vi "WS1021 MEMS Only 24DUT CV Sweep Header BCBE.vi"(8 "Error In":errorcluster) -> (0 "Error Out":errorcluster, 3 "Name Calculated Header":string[](array[string]))   [LabVIEW 2017]
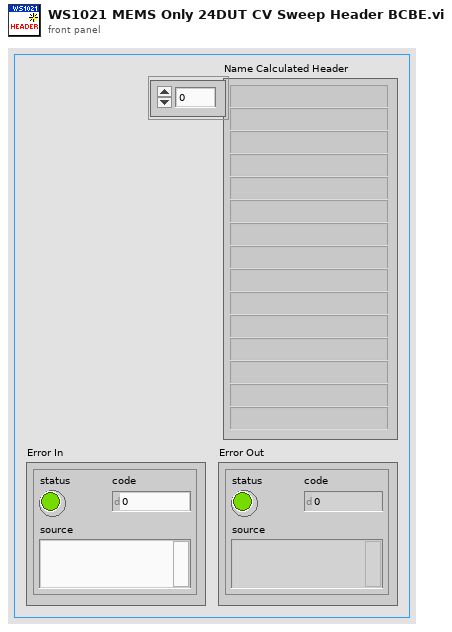
[diagram p1: front panel]
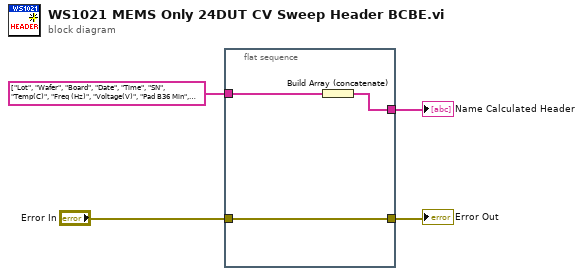
[diagram p0: block diagram]
diagram:
  n1 = flat-sequence {
    tunnel: "Error In" -> [w7]
    tunnel: [w7] -> w4
    tunnel: string[] ["Lot", "Wafer", "Board", "Date", "Time", "SN", "Temp(C)", "Freq (Hz)", "Voltage(V)", "Pad B36 Min", "B36 Min (fF)", "Pad B36 Max", "B36 Max (fF)", "Pad B25 Min", "B25 Min (fF)", "Pad B25 Max", "B25 Max (fF)", "Pad 12 Beams Min", "12 Beams Min (fF)", "Pad 12 Beams Max", "12 Beams Max (fF)", "B36 Min_DCap (fF)", "B36 Max_DCap (fF)", "B25 Min_DCap (fF)", "B25 Max_DCap (fF)", "12 Beams Min_DCap (fF)", "12 Beams Max_DCap (fF)", "Command", "Test Program"] -> [w6]
    tunnel: [w5] -> w2
    frame #0 {
      n2 = Build Array (concatenate)(w6) -> (w5:string[])
    }
  }
  "Name Calculated Header" <- w2
  "Error Out" <- w4
